vi "Generate GraphViz Mapping File.vi"(7 "supported colors":string[](array[string])=["dodgerblue", "cadetblue1", "darkgoldenrod1", "gainsboro"], 8 "Show Unmapped Channels?":bool=TRUE, 9 "Show Tag Labels?":bool=TRUE, 10 "Modules Configurations":refnum<class "TBM module configuration.lvclass">[](array[class]), 11 "engine configuration in":refnum<class "engine configuration.lvclass">) -> (3 "output to graphviz":string)   [LabVIEW 2013, in "GraphViz Mapping Visualizer.lvlib"]
uses:
  GraphViz Mapping Visualizer.lvlib
  <vilib>/NI/Tag Bus Module Framework/module configuration/TBM module configuration.lvclass
  <vilib>/NI/Module Execution Interface/Engine Configuration/engine configuration.lvclass
  Channel to Port Pair.ctl
  <vilib>/NI/Tag Bus/tag/tag descriptor.lvclass/tag descriptor.ctl
  <vilib>/NI/Tag Bus Module Framework/channel/channel classification.ctl
  <vilib>/NI/Tag Bus/tag/read tag name.vi
  <vilib>/NI/Tag Bus/tag/read data type.vi
  <vilib>/NI/Tag Bus Module Framework/channel/TBM channel.lvclass
  Configuration Editor/Classes/Engine Mappings/Engine Mappings.lvclass
  <vilib>/NI/Tag Bus/tag/tag descriptor.lvclass
panel:
  in  "file path (use dialog)":path
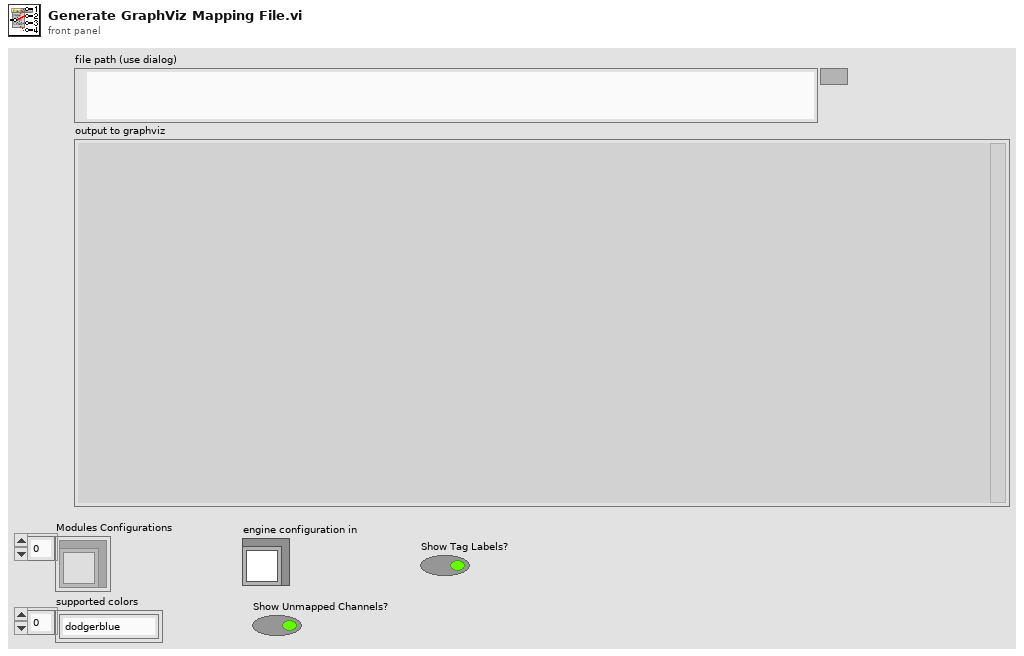
[diagram p1: front panel]
types:
  T1 = typedef "GraphViz Mapping Visualizer.lvlib/Channel to Port Pair.ctl" = cluster{"Channel Name":string, "Node:Port":string}
  T2 = typedef "PL Framework Configuration Tool.lvlib/Engine Mappings.lvclass/module information.ctl" = cluster{"display name":string, "instance id":string, "channels":refnum<class "TBM channel.lvclass">[]}
  T3 = typedef "TBM channel.lvclass/channel classification.ctl" = enum16{"input data", "output data", "processing parameter", "processing result"}
  T4 = typedef "engine configuration.lvclass/Tag Info.ctl" = cluster{"Tag":refnum<class "tag descriptor.lvclass">, "Writer Module":string, "Writer Channel":string, "Readers":cluster{"module":string, "channel":string}[], "Owning ID":string}
  T5 = typedef "tag bus.lvlib/tag descriptor.lvclass/Data Type.ctl" = enum16{"Double", "Single", "I64", "I32", "I16", "I8", "U64", "U32", "U16", "U8", "Boolean", "String", "Array of Double", "Array of Single", "Array of I64", "Array of I32", "Array of I16", "Array of I8", "Array of U64", "Array of U32", "Array of U16", "Array of U8", "Array of Boolean", "Array of String"}
  T6 = enum16{"open", "replace", "create", "open or create", "replace or create", "replace or create with confirmation"}
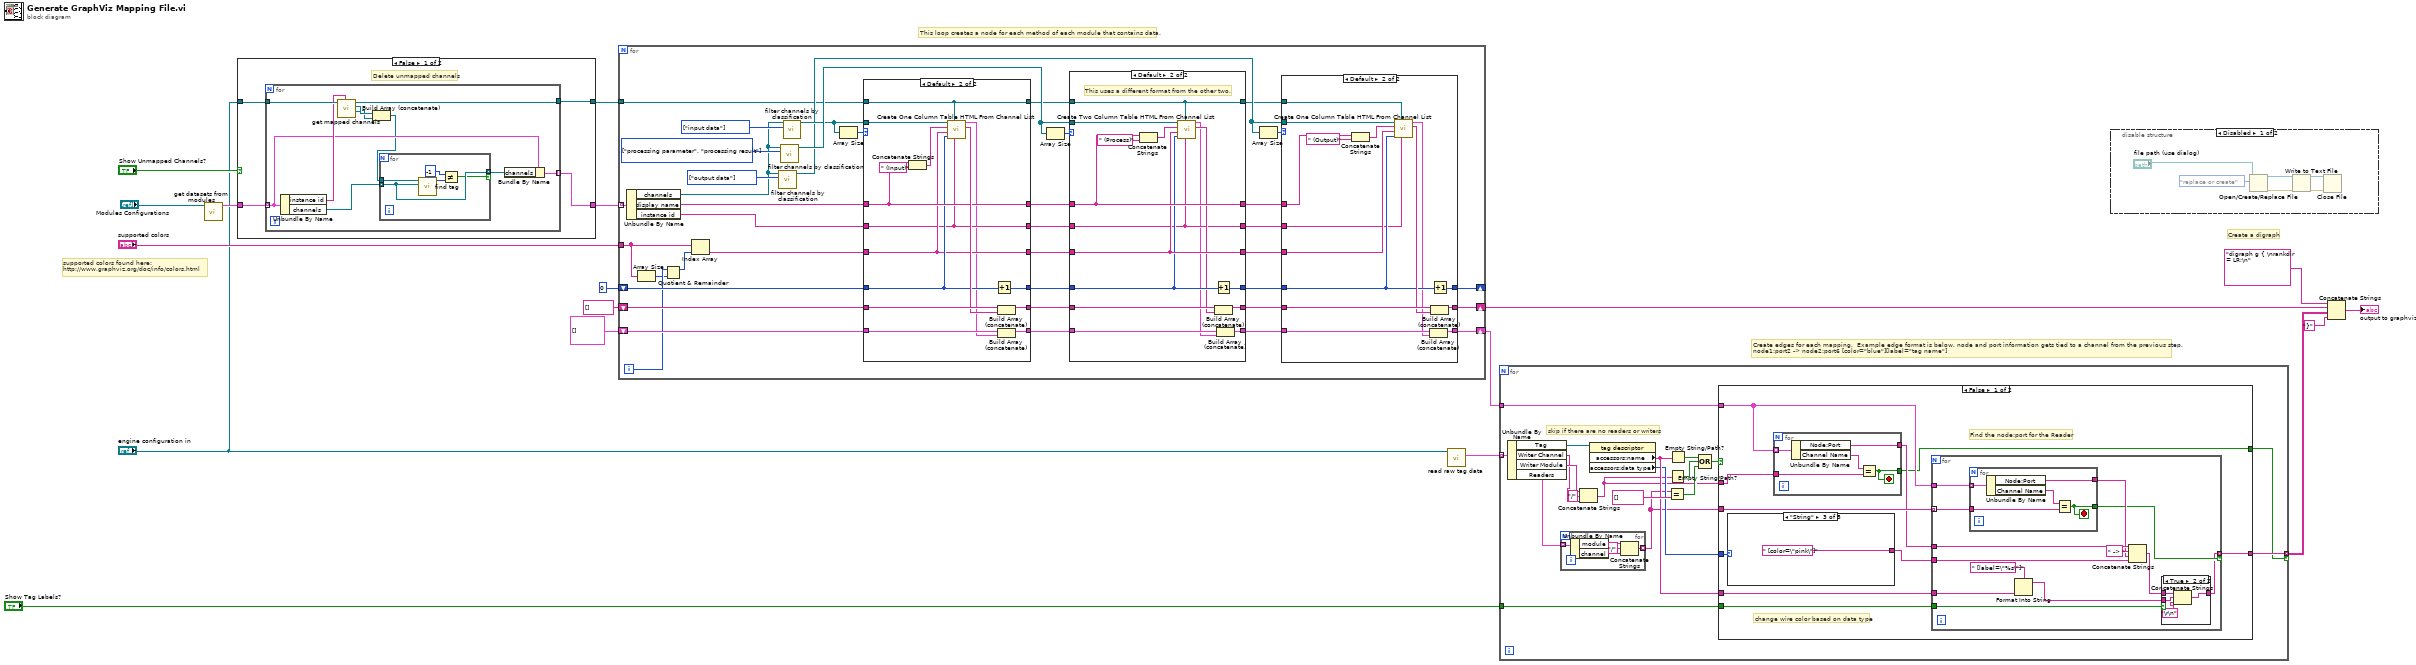
[diagram p0: block diagram]
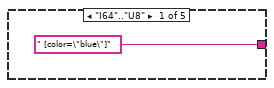
[diagram p3: hidden frame]
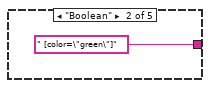
[diagram p4: hidden frame]
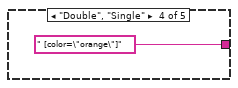
[diagram p5: hidden frame]
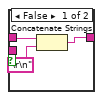
[diagram p7: hidden frame]
diagram:
  # "This loop creates a node for each method of each module that contains data."
  # "Create a digraph"
  # "supported colors found here:\nhttp://www.graphviz.org/doc/info/colors.html"
  # "Create edges for each mapping.  Example edge format is below. node and port information gets tied to a channel from the previous step.\nnode1:port2 -> node2:port6 [color=\"blue\"][label=\"tag name\"]"
  n1 = call "get datasets from modules.vi"("Modules Configurations"="Modules Configurations") -> ("module datasets"=w6:T2[])  [unwired: 9 in, 1 out]
  n2 = case shown="False" "Show Unmapped Channels?" {
    tunnel: w6 -> [w22 w39]
    tunnel: [w19 w39] -> w5
    tunnel: "engine configuration in" -> [w21 w38]
    tunnel: [w20 w38] -> w4
    frame False {
      # "Delete unmapped channels"
      n3 = for {
        tunnel: w22 -> [w28] mode=indexing
        tunnel: w21 -> [w32]
        tunnel: [w31] -> w20
        tunnel: [w26] -> w19 mode=indexing
        n4 = Unbundle By Name(w28) -> ("instance id"=w30:string, "channels"=w29:refnum<class "TBM channel.lvclass">[])
        n5 = call <vilib>:"get mapped channels.vi"("owner"=w30, "engine configuration in"=w32) -> ("write channels"=w24:refnum<class "TBM channel.lvclass">[], "read channels"=w25:refnum<class "TBM channel.lvclass">[], "engine configuration out"=w31:refnum<class "engine configuration.lvclass">)  [unwired: 5 in, 2 out]
        n6 = Build Array (concatenate)(w25, w24) -> (w23:refnum<class "TBM channel.lvclass">[])
        n7 = for {
          tunnel: w23 -> [w35]
          tunnel: w29 -> [w34] mode=indexing
          tunnel: [w34] -> w27 mode=indexing if=w33
          n8 = call <vilib>:"find tag.vi"("tag"=w34, "tags in"=w35) -> ("index"=w36:i32)  [unwired: 9 in]
          n9 = Not Equal?(x=-1, y=w36) -> (x != y?=w33:bool)
        }
        n10 = Bundle By Name(cluster=w28, "channels"=w27) -> (w26:T2)
      }
    }
    frame True {
    }
  }
  n11 = for {
    tunnel: w5 -> [w78] mode=indexing
    shift-right: [w65] -> w13
    shift-left: string[] [] -> [w76]
    shift-right: [w64] -> _
    shift-left: 0 -> [w72]
    shift-right: [w61] -> w10
    shift-left: T1[] [] -> [w62]
    tunnel: "supported colors" -> [w56]
    tunnel: w4 -> [w42]
    i -> [w55]
    w45 = T3[] [enum."output data"] items=["input data", "output data", "processing parameter", "processing result"] ("allowed classifications")
    w48 = T3[] [enum."processing parameter", enum."processing result"] items=["input data", "output data", "processing parameter", "processing result"] ("allowed classifications")
    w49 = T3[] [enum."input data"] items=["input data", "output data", "processing parameter", "processing result"] ("allowed classifications")
    n12 = Unbundle By Name(w78) -> ("channels"=w44:refnum<class "TBM channel.lvclass">[], "display name"=w73:string, "instance id"=w63:string)
    n13 = Array Size(array=w56) -> (size(s)=w54:i32)
    n14 = Quotient & Remainder(x=w55, y=w54) -> (x-y*floor(x/y)=w53:i32)  [unwired: 1 out]
    n15 = Index Array(array=w56, index=w53) -> (element=w52:string)
    n16 = call <vilib>:"filter channels by classification.vi"("allowed classifications"=w45, "channels in"=w44) -> ("channels out"=w43:refnum<class "TBM channel.lvclass">[])  [unwired: 9 in]
    n17 = call <vilib>:"filter channels by classification.vi"("allowed classifications"=w48, "channels in"=w44) -> ("channels out"=w47:refnum<class "TBM channel.lvclass">[])  [unwired: 9 in]
    n18 = call <vilib>:"filter channels by classification.vi"("allowed classifications"=w49, "channels in"=w44) -> ("channels out"=w46:refnum<class "TBM channel.lvclass">[])  [unwired: 9 in]
    n19 = Array Size(array=w46) -> (size(s)=w77:i32)
    n20 = case shown="Default" w77 {
      tunnel: w46 -> [_ w131]
      tunnel: [w125 w140] -> w75
      tunnel: w76 -> [w125 w139]
      tunnel: w73 -> [w123 w134]
      tunnel: w72 -> [w124 w132]
      tunnel: [w124 w136] -> w70
      tunnel: [w123 w134] -> w71
      tunnel: w63 -> [w121 w128]
      tunnel: w62 -> [w122 w133]
      tunnel: [w122 w130] -> w59
      tunnel: [w121 w128] -> w58
      tunnel: w52 -> [w120 w129]
      tunnel: [w120 w129] -> w51
      tunnel: w42 -> [w119 w126]
      tunnel: [w119 w126] -> w41
      frame 0 {
        # "don't create a node if there are no channels of that type"
      }
      frame Default {
        n21 = Concatenate Strings(w134, " (Input)" ("string")) -> (w137:string)
        n22 = call "Create One Column Table HTML From Channel List.vi"("Instance ID"=w128, "engine configuration in"=w126, "Node#"=w132, "Color"=w129, "Title"=w137, "Channels"=w131) -> ("Table HTML"=w135:string, "Channel and Node Pairs"=w127:T1[])  [unwired: 4 in]
        n23 = Increment(x=w132) -> (x+1=w136:i32)
        n24 = Build Array (concatenate)(w139, w135) -> (w140:string[])
        n25 = Build Array (concatenate)(w133, w127) -> (w130:T1[])
      }
    }
    n26 = Array Size(array=w47) -> (size(s)=w74:i32)
    n27 = case shown="Default" w74 {
      tunnel: w47 -> [_ w111]
      tunnel: [w103 w118] -> w68
      tunnel: w75 -> [w103 w117]
      tunnel: w71 -> [w101 w114]
      tunnel: w70 -> [w102 w108]
      tunnel: [w102 w115] -> w69
      tunnel: [w101 w114] -> w67
      tunnel: [w100 w113] -> w60
      tunnel: w59 -> [w100 w112]
      tunnel: w58 -> [w99 w106]
      tunnel: [w99 w106] -> w57
      tunnel: w51 -> [w98 w109]
      tunnel: [w98 w109] -> w50
      tunnel: w41 -> [w97 w104]
      tunnel: [w97 w104] -> w40
      frame 0 {
        # "don't create a node if there are no channels of that type"
      }
      frame Default {
        # "This uses a different format from the other two."
        n28 = Concatenate Strings(w114, " (Process)" ("string")) -> (w110:string)
        n29 = call "Create Two Column Table HTML From Channel List.vi"("Instance ID"=w106, "engine configuration in"=w104, "Node#"=w108, "Color"=w109, "Title"=w110, "Channels"=w111) -> ("Table HTML"=w107:string, "Channel and Node Pairs"=w105:T1[])  [unwired: 4 in]
        n30 = Increment(x=w108) -> (x+1=w115:i32)
        n31 = Build Array (concatenate)(w117, w107) -> (w118:string[])
        n32 = Build Array (concatenate)(w112, w105) -> (w113:T1[])
      }
    }
    n33 = Array Size(array=w43) -> (size(s)=w66:i32)
    n34 = case shown="Default" w66 {
      tunnel: w43 -> [_ w87]
      tunnel: [w81 w96] -> w65
      tunnel: w68 -> [w81 w95]
      tunnel: w67 -> [_ w93]
      tunnel: w69 -> [w80 w86]
      tunnel: [w80 w90] -> w64
      tunnel: [w79 w89] -> w61
      tunnel: w60 -> [w79 w88]
      tunnel: w57 -> [_ w83]
      tunnel: w50 -> [_ w85]
      tunnel: w40 -> [_ w82]
      frame 0 {
        # "don't create a node if there are no channels of that type"
      }
      frame Default {
        n35 = Concatenate Strings(w93, " (Output)" ("string")) -> (w92:string)
        n36 = call "Create One Column Table HTML From Channel List.vi"("Instance ID"=w83, "engine configuration in"=w82, "Node#"=w86, "Color"=w85, "Title"=w92, "Channels"=w87) -> ("Table HTML"=w91:string, "Channel and Node Pairs"=w84:T1[])  [unwired: 4 in]
        n37 = Build Array (concatenate)(w88, w84) -> (w89:T1[])
        n38 = Build Array (concatenate)(w95, w91) -> (w96:string[])
        n39 = Increment(x=w86) -> (x+1=w90:i32)
      }
    }
  }
  n40 = call <vilib>:"read raw tag data.vi"("engine configuration in"="engine configuration in") -> ("raw tag data"=w1:T4[])  [unwired: 8 in, 2 out]
  n41 = for {
    tunnel: w1 -> [w159] mode=indexing
    tunnel: w10 -> [w152]
    tunnel: [w150] -> w9 mode=indexing if=w149
    tunnel: "Show Tag Labels?" -> [w148]
    # "skip if there are no readers or writers"
    n42 = Unbundle By Name(w159) -> ("Tag"=w158:refnum<class "tag descriptor.lvclass">, "Writer Channel"=w142:string, "Writer Module"=w143:string, "Readers"=w145:cluster{"module":string, "channel":string}[])
    n43 = for {
      tunnel: w145 -> [w164] mode=indexing
      tunnel: [w160] -> w146 mode=indexing
      n44 = Unbundle By Name(w164) -> ("module"=w163:string, "channel"=w162:string)
      n45 = Concatenate Strings(w163, "/" ("string"), w162) -> (w160:string)
    }
    n46 = Concatenate Strings(w143, "/" ("string"), w142) -> (w141:string)
    n47 = property class="tag descriptor"(reference=w158) -> ("accessors:name"=w151:string, "accessors:data type"=w147:T5)  [unwired: 1 in, 2 out]
    n48 = Equal?(x=w146, y=string[] []) -> (x = y?=w154:bool)
    n49 = Empty String/Path?(string/path=w141) -> (empty?=w155:bool)
    n50 = Empty String/Path?(string/path=w151) -> (empty?=w156:bool)
    n51 = Compound Arithmetic op=OR(w156, w155, w154) -> (w153:bool)
    n52 = case shown="False" w153 {
      tunnel: w152 -> [w173 _]
      tunnel: w146 -> [w174 _]
      tunnel: w141 -> [w172 _]
      tunnel: w151 -> [w170 _]
      tunnel: [w169 _] -> w150
      tunnel: [w168 _] -> w149
      tunnel: w148 -> [w167 _]
      tunnel: w147 -> [w166 _]
      frame False {
        # "Find the node:port for the Reader"
        # "change wire color based on data type"
        n53 = case shown="\"String\"" w166 {
          tunnel: [" [color=\"blue\"]" ("string") " [color=\"green\"]" ("string") " [color=\"pink\"]" ("string") " [color=\"orange\"]" ("string") _] -> w165
          frame "I64".."U8" {
          }
          frame "Boolean" {
          }
          frame "String" {
          }
          frame "Double", "Single" {
          }
          frame Default {
          }
        }
        n54 = for {
          tunnel: w172 -> [w181]
          tunnel: w173 -> [w183] mode=indexing
          tunnel: [w180] -> w168
          tunnel: [w179] -> w171
          stop <- w180 stop-if-true
          n55 = Unbundle By Name(w183) -> ("Node:Port"=w179:string, "Channel Name"=w182:string)
          n56 = Equal?(x=w182, y=w181) -> (x = y?=w180:bool)
        }
        n57 = for {
          tunnel: w174 -> [w196] mode=indexing
          tunnel: w173 -> [w195]
          tunnel: w171 -> [w194]
          tunnel: w170 -> [w191]
          tunnel: [w185] -> w169 mode=indexing if=w189
          tunnel: w167 -> [w188]
          tunnel: w165 -> [w184]
          n58 = for {
            tunnel: w196 -> [w206]
            tunnel: w195 -> [w208] mode=indexing
            tunnel: [w205] -> w189
            tunnel: [w204] -> w190
            stop <- w205 stop-if-true
            n59 = Unbundle By Name(w208) -> ("Node:Port"=w204:string, "Channel Name"=w207:string)
            n60 = Equal?(x=w207, y=w206) -> (x = y?=w205:bool)
          }
          n61 = Format Into String(format string=" [label=\"%s\"]" ("string"), w191) -> (resulting string=w187:string)  [unwired: 2 in, 1 out]
          n62 = Concatenate Strings(w194, " -> " ("string"), w190, w184) -> (w186:string)
          n63 = case shown="True" w188 {
            tunnel: w187 -> [_ w202]
            tunnel: w186 -> [w199 w203]
            tunnel: [w197 w201] -> w185
            frame False {
              n64 = Concatenate Strings(w199, "\r\n") -> (w197:string)
            }
            frame True {
              n65 = Concatenate Strings(w203, w202, "\r\n") -> (w201:string)
            }
          }
        }
      }
      frame True {
      }
    }
  }
  n66 = disable-structure shown="Disabled" {
    frame Disabled {
      n67 = Open/Create/Replace File(file path (use dialog)="file path (use dialog)", operation (0:open)=T6."replace or create") -> (refnum out=w210:refnum<file>, error out=w209:errorcluster)  [unwired: 4 in, 1 out]
      n68 = Write to Text File(file (use dialog)=w210, error in=w209) -> (refnum out=w211:refnum<file>, error out=w212:errorcluster)  [unwired: 2 in, 1 out]
      n69 = Close File(refnum=w211, error in=w212) -> ()  [unwired: 2 out]
    }
    frame Enabled {
    }
  }
  n70 = Concatenate Strings("digraph g { \nrankdir = LR;\n", w13, w9, "}") -> (→"output to graphviz":string)
